vi "ITM10_Status.vi"() -> (1 "n_ng":u8, 2 "values":T1)   [LabVIEW 2019]
uses:
  ITM10_Global.vi
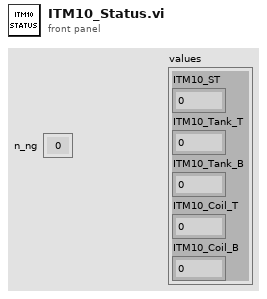
[diagram p1: front panel]
types:
  T1 = cluster{"ITM10_ST":u32, "ITM10_Tank_T":dbl, "ITM10_Tank_B":dbl, "ITM10_Coil_T":dbl, "ITM10_Coil_B":dbl}
  T2 = enum32{"Bad", "Idle", "Run top level", "Running"}
  T3 = cluster{"MKS670_1000_ST":u32, "ITM10_Tank_T":dbl, "ITM10_Tank_B":dbl, "ITM10_Coil_T":dbl, "ITM10_Coil_B":dbl}
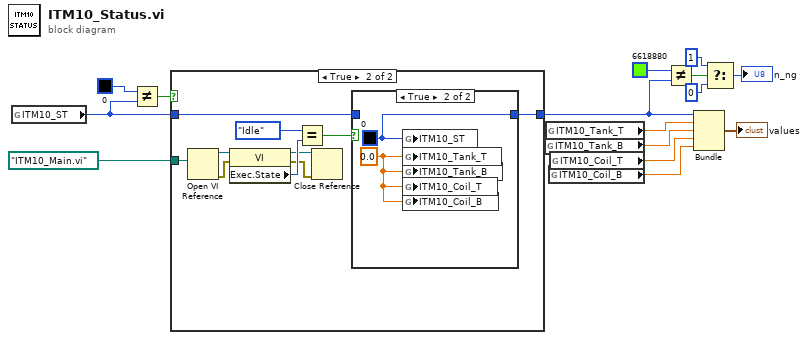
[diagram p0: block diagram]
diagram:
  n1 = global read "ITM10_Global.vi" "ITM10_ST"() -> (w6:u32)
  n2 = Not Equal?(x=u32 0 ("MKS670_1000_ST 2"), y=w6) -> (x != y?=w15:bool)
  n3 = case shown="True" w15 {
    tunnel: w6 -> [w16 w18]
    tunnel: [w16 w17] -> w12
    tunnel: path "ITM10_Main.vi" ("vi path") -> [_ w19]
    frame False {
    }
    frame True {
      n4 = Open VI Reference(vi path=w19) -> (vi reference=w26:refnum<vi>, error out=w25:errorcluster)  [unwired: 5 in]
      n5 = property class="VI"(reference=w26, error in=w25) -> (reference out=w21:refnum<vi>, error out=w20:errorcluster, "Exec.State"=w23:T2)
      n6 = Equal?(x=T2."Idle" ("Execution:State"), y=w23) -> (x = y?=w24:bool)
      n7 = Close Reference(reference=w21, error in (no error)=w20) -> ()  [unwired: 1 out]
      n8 = case shown="True" w24 {
        tunnel: w18 -> [w27 _]
        tunnel: [w27 w29] -> w17
        frame False {
        }
        frame True {
          w28 = 0.0 ("MKS670_1000_P")
          w29 = u32 0 ("MKS670_1000_ST")
          n9 = global write "ITM10_Global.vi" "ITM10_ST"(w29) -> ()
          n10 = global write "ITM10_Global.vi" "ITM10_Tank_T"(w28) -> ()
          n11 = global write "ITM10_Global.vi" "ITM10_Tank_B"(w28) -> ()
          n12 = global write "ITM10_Global.vi" "ITM10_Coil_T"(w28) -> ()
          n13 = global write "ITM10_Global.vi" "ITM10_Coil_B"(w28) -> ()
        }
      }
    }
  }
  n14 = global read "ITM10_Global.vi" "ITM10_Tank_B"() -> (w4:dbl)
  n15 = global read "ITM10_Global.vi" "ITM10_Tank_T"() -> (w5:dbl)
  n16 = global read "ITM10_Global.vi" "ITM10_Coil_B"() -> (w2:dbl)
  n17 = global read "ITM10_Global.vi" "ITM10_Coil_T"() -> (w3:dbl)
  n18 = Not Equal?(x=u32 6618880 ("MKS670_1000_ST 2"), y=w12) -> (x != y?=w10:bool)
  n19 = Bundle("MKS670_1000_ST"=w12, "ITM10_Tank_T"=w5, "ITM10_Tank_B"=w4, "ITM10_Coil_T"=w3, "ITM10_Coil_B"=w2) -> (→"values":T3)  [unwired: 1 in]
  n20 = Select(t=u8 1 ("n_ng"), s=w10, f=u8 0 ("n_ng")) -> (s? t:f=→"n_ng":u8)
